vi "ArdnoMix.vi"(0 "LINX Resource":T1={"IO"=enum."Remote", "Interface"=enum."Serial", "LINX Device Config"={"Interface"=enum."Serial", "COM Port"="COM13", "TCP Configuration"={"IP Address"="", "Port"=0}, "Device Family"=1, "Device ID"=1, "Device Name"="myRIO-1900", "TCP Ref"=refnum, "Channels"={"DI"=[0, 1, 2, 3, 4, 5, 6, 7, 8, 9, 10, 11, 12, 13, 14, 15, 16, 17, 18, 19, 20, 21, 22, 23, 24, 25, 26, 27, 28, 29, 30, 31, 32, 33, 34, 35, 36, 37, 38, 39, 40, 41, 42, 43, 44, 45, 46], "DO"=[0, 1, 2, 3, 4, 5, 6, 7, 8, 9, 10, 11, 12, 13, 14, 15, 16, 17, 18, 19, 20, 21, 22, 23, 24, 25, 26, 27, 28, 29, 30, 31, 32, 33, 34, 35, 36, 37, 38, 39, 40, 41, 42, 43, 44, 45, 46], "AI"=[0, 1, 2, 3, 4, 5, 6, 7, 8, 9, 10, 11], "AO"=[], "PWM"=[3, 5, 6, 9, 10], "QE"=[], "UART"=[0, 1], "I2C 2"=[0], "SPI"=[0], "CAN"=[], "Servo"=[], "AI Ref (V)"=0.0, "AI Resolution (Bits)"=0, "AO Ref (V)"=0.0, "AO Resolution (Bits)"=0}}}, 1 "Mix Cycles":i32, 2 "Single/\nMultiring?":u16(ring) items=["8-Ring", "OneRing"], 3 "error in (no error)":errorcluster, 4 "Mix Frequency":i32=4) -> (5 "LINX Resource out":T1, 6 "Elapsed [ms]":u32, 7 "ValveStates":bool[](array[boolean]), 8 "error out":errorcluster)   [LabVIEW 2018, in "Arduino.lvlib"]
uses:
  Arduino.lvlib
  <vilib>/MakerHub/LINX/Private/Type Defs/LINX Ref.ctl
  <vilib>/MakerHub/LINX/Private/Type Defs/Platform.ctl
  <vilib>/MakerHub/LINX/Private/Type Defs/Interface.ctl
  <vilib>/MakerHub/LINX/Private/Device/Type Defs/LINX Device Config.ctl
  <vilib>/MakerHub/LINX/Private/Device/Type Defs/TCP Config.ctl
  <vilib>/MakerHub/LINX/Private/Device/Type Defs/Channels.ctl
  <vilib>/MakerHub/LINX/Public/Peripherals/Digital/Digital Write N Chans.vi
  <vilib>/MakerHub/LINX/Private/Local IO/LinxDigitalWrite.vi
  <vilib>/MakerHub/LINX/Public/Utilities/Check Channel.vi
  <vilib>/MakerHub/LINX/Private/Utilties/Generate Error.vi
  <vilib>/MakerHub/LINX/LMH-LINX.lvlib
  <vilib>/MakerHub/LINX/Private/Device/Device.lvlib
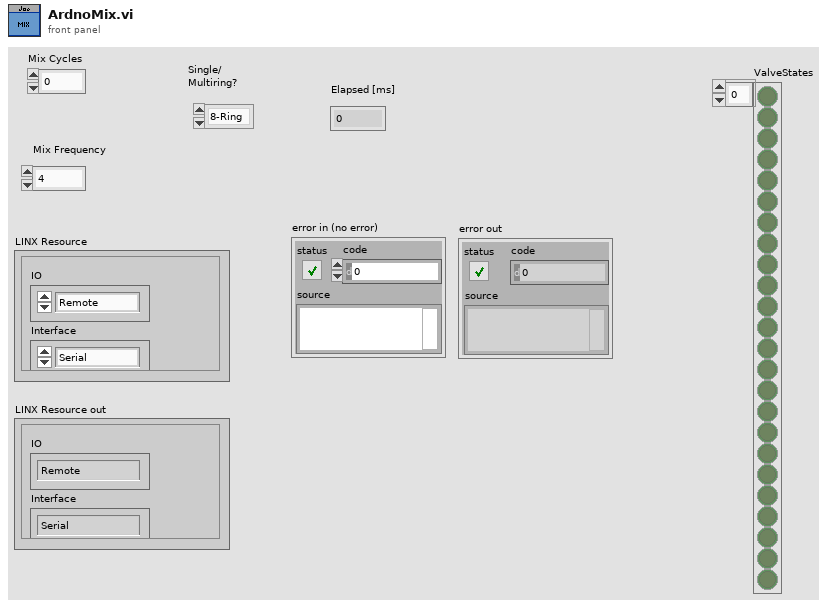
[diagram p1: front panel]
types:
  T1 = typedef "LMH-LINX.lvlib/LINX Ref.ctl" = cluster{"IO":T2, "Interface":T3, "LINX Device Config":T4}
  T2 = typedef "LMH-LINX.lvlib/Platform.ctl" = enum16{"Remote", "Local"}
  T3 = typedef "LMH-LINX.lvlib/Interface.ctl" = enum16{"Serial", "TCP"}
  T4 = typedef "LMH-LINX.lvlib/Device.lvlib/LINX Device Config.ctl" = cluster{"Interface":T3, "COM Port":refnum<visa-resource-name>, "TCP Configuration":T5, "Device Family":u8, "Device ID":u8, "Device Name":string, "TCP Ref":refnum<k5>, "Channels":T6}
  T5 = typedef "LMH-LINX.lvlib/Device.lvlib/TCP Config.ctl" = cluster{"IP Address":string, "Port":u16}
  T6 = typedef "LMH-LINX.lvlib/Channels.ctl" = cluster{"DI":u8[], "DO":u8[], "AI":u8[], "AO":u8[], "PWM":u8[], "QE":u8[], "UART":u8[], "I2C 2":u8[], "SPI":u8[], "CAN":u8[], "Servo":u8[], "AI Ref (V)":dbl, "AI Resolution (Bits)":u8, "AO Ref (V)":dbl, "AO Resolution (Bits)":u8}
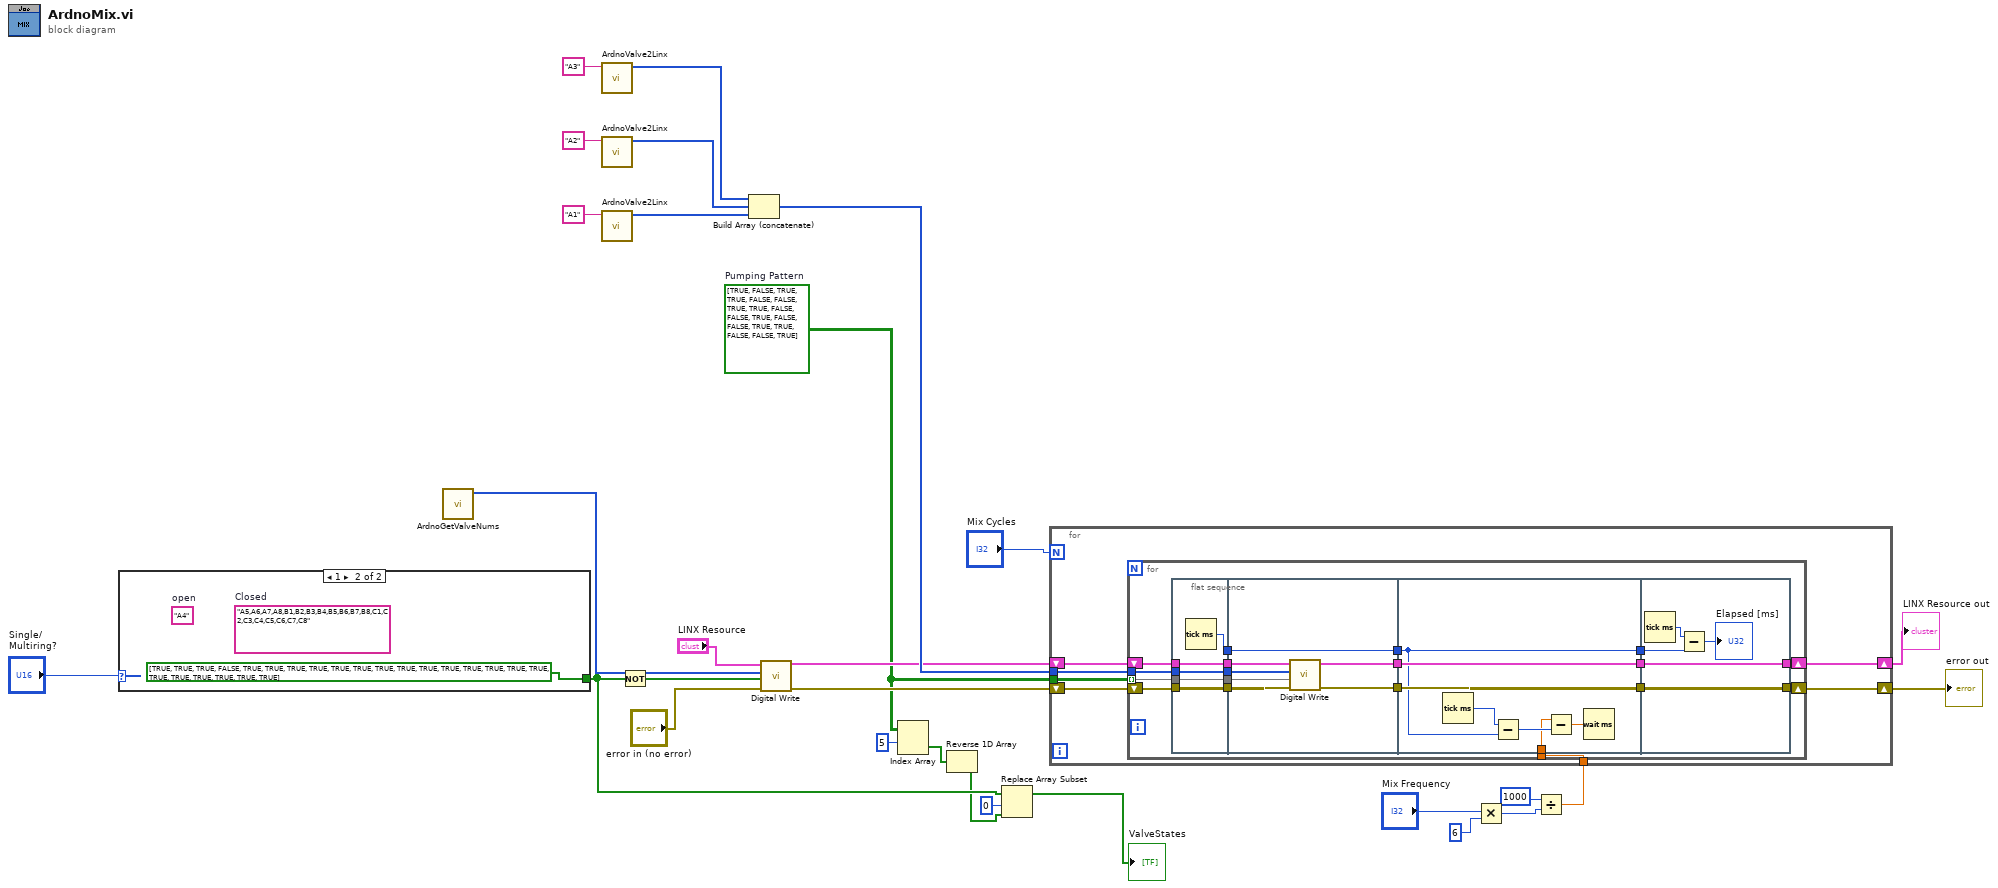
[diagram p0: block diagram]
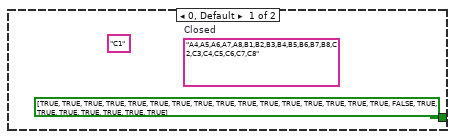
[diagram p2: hidden frame]
diagram:
  w8 = bool[][] [[TRUE, FALSE, TRUE], [TRUE, FALSE, FALSE], [TRUE, TRUE, FALSE], [FALSE, TRUE, FALSE], [FALSE, TRUE, TRUE], [FALSE, FALSE, TRUE]]  # Pumping Pattern
  n1 = case shown="1" "Single/\nMultiring?" {
    tunnel: [bool[] [TRUE, TRUE, TRUE, TRUE, TRUE, TRUE, TRUE, TRUE, TRUE, TRUE, TRUE, TRUE, TRUE, TRUE, TRUE, TRUE, FALSE, TRUE, TRUE, TRUE, TRUE, TRUE, TRUE, TRUE] bool[] [TRUE, TRUE, TRUE, FALSE, TRUE, TRUE, TRUE, TRUE, TRUE, TRUE, TRUE, TRUE, TRUE, TRUE, TRUE, TRUE, TRUE, TRUE, TRUE, TRUE, TRUE, TRUE, TRUE, TRUE]] -> w6
    frame 0, Default {
      (unwired) "A4,A5,A6,A7,A8,B1,B2,B3,B4,B5,B6,B7,B8,C2,C3,C4,C5,C6,C7,C8"  # Closed
      (unwired) "C1" ("open")
    }
    frame 1 {
      (unwired) "A5,A6,A7,A8,B1,B2,B3,B4,B5,B6,B7,B8,C1,C2,C3,C4,C5,C6,C7,C8"  # Closed
      (unwired) "A4"  # open
    }
  }
  n2 = call "ArdnoGetValveNums.vi"() -> ("Array"=w9:i32[])  [unwired: 11 in]
  n3 = call "ArdnoValve2Linx.vi"("Valve (A1-C8),\n comma separated"="A3") -> ("Linx Port"=w26:i32[])  [unwired: 8 in, 2 out]
  n4 = call "ArdnoValve2Linx.vi"("Valve (A1-C8),\n comma separated"="A2") -> ("Linx Port"=w25:i32[])  [unwired: 8 in, 2 out]
  n5 = call "ArdnoValve2Linx.vi"("Valve (A1-C8),\n comma separated"="A1") -> ("Linx Port"=w24:i32[])  [unwired: 8 in, 2 out]
  n6 = Not(x=w6) -> (.not. x?=w1:bool[])
  n7 = Build Array (concatenate)(w26, w25, w24) -> (w23:i32[])
  n8 = call-poly <vilib>:"Digital Write.vi"("Error In"="error in (no error)", "Values"=w1, "DO Channels"=w9, "LINX Resource"="LINX Resource") -> ("Error Out"=w18:errorcluster, "LINX Resource"=w19:T1)  [unwired: 6 in]
  n9 = Index Array(array=w8, index (row)=5) -> (element=w3:bool[])  [unwired: 1 in]
  n10 = Reverse 1D Array(array=w3) -> (reversed array=w2:bool[])
  n11 = Replace Array Subset(array=w6, new element=w2, index=0) -> (→"ValveStates":bool[])
  n12 = Multiply(x="Mix Frequency", y=6) -> (x*y=w15:i32)
  n13 = Divide(x=u32 1000, y=w15) -> (x/y=w11:dbl)
  n14 = for {
    N: "Mix Cycles" -> [_]
    tunnel: w23 -> [w37]
    tunnel: w8 -> [w35]
    shift-right: [w33] -> w22
    shift-left: w19 -> [w36]
    shift-right: [w32] -> w21
    shift-left: w18 -> [w34]
    tunnel: w11 -> [w38]
    n15 = for {
      tunnel: w35 -> [w51] mode=indexing
      tunnel: w37 -> [w54]
      shift-right: [w53] -> w33
      shift-left: w36 -> [w56]
      shift-right: [w52] -> w32
      shift-left: w34 -> [w55]
      tunnel: w38 -> [w42]
      n16 = flat-sequence {
        tunnel: w51 -> [w58]
        tunnel: w54 -> [w59]
        tunnel: w55 -> [w60]
        tunnel: w56 -> [w61]
        tunnel: [w61] -> w50
        tunnel: [w60] -> w49
        tunnel: [w59] -> w48
        tunnel: [w58] -> w47
        tunnel: [w57] -> w46
        tunnel: [w65] -> w41
        tunnel: [w64] -> w40
        tunnel: w50 -> [w68]
        tunnel: w49 -> [w67]
        tunnel: w48 -> [w66]
        tunnel: w47 -> [w63]
        tunnel: w46 -> [w62]
        tunnel: [w62] -> w39
        tunnel: w41 -> [w75]
        tunnel: w40 -> [w74]
        tunnel: w39 -> [w72]
        tunnel: [w75] -> w45
        tunnel: [w74] -> w44
        tunnel: [w72] -> w43
        tunnel: w42 -> [w69]
        tunnel: [w79] -> w52
        tunnel: [w80] -> w53
        tunnel: w45 -> [w80]
        tunnel: w44 -> [w79]
        tunnel: w43 -> [w76]
        frame #0 {
          n17 = Tick Count (ms)() -> (millisecond timer value=w57:u32)
        }
        frame #1 {
          n18 = call-poly <vilib>:"Digital Write.vi"("Error In"=w67, "Values"=w63, "DO Channels"=w66, "LINX Resource"=w68) -> ("Error Out"=w64:errorcluster, "LINX Resource"=w65:T1)  [unwired: 6 in]
        }
        frame #2 {
          n19 = Tick Count (ms)() -> (millisecond timer value=w73:u32)
          n20 = Subtract(x=w73, y=w72) -> (x-y=w71:u32)
          n21 = Subtract(x=w69, y=w71) -> (x-y=w70:dbl)
          n22 = Wait (ms)(milliseconds to wait=w70) -> ()  [unwired: 1 out]
        }
        frame #3 {
          n23 = Tick Count (ms)() -> (millisecond timer value=w77:u32)
          n24 = Subtract(x=w77, y=w76) -> (x-y=→"Elapsed [ms]":u32)
        }
      }
    }
  }
  "error out" <- w21
  "LINX Resource out" <- w22
